vi "get_numbers_in_string.vi"(3 "String":string="one 2 -3 4.0 5.5") -> (0 "Total numbers":i32, 1 "Extracted Numbers":dbl[](array[numeric]) format="%#.6g")   [LabVIEW 2018]
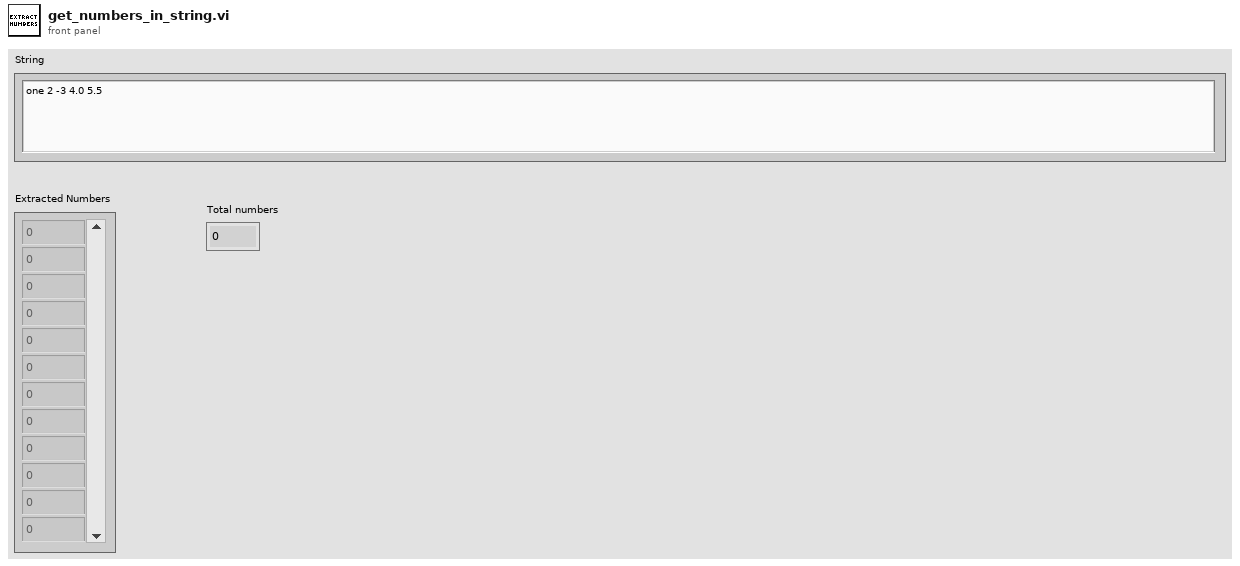
[diagram p1: front panel]
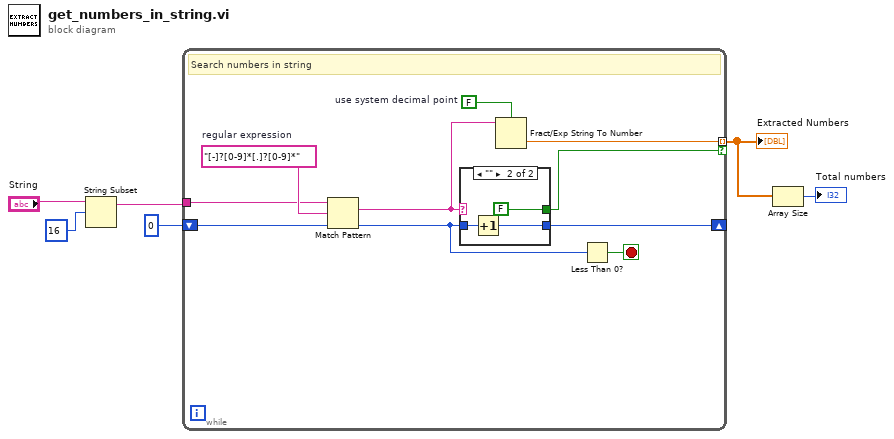
[diagram p0: block diagram]
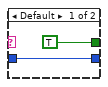
[diagram p2: hidden frame]
diagram:
  n1 = String Subset(string="String", offset (0)=16) -> (substring=w2:string)  [unwired: 1 in]
  n2 = while {
    shift-left: 0 -> [w12]
    shift-right: [w7] -> _
    tunnel: [w16] -> w5 mode=indexing if=w9
    tunnel: w2 -> [w11]
    stop <- w15 stop-if-true
    w14 = FALSE  # use system decimal point
    w13 = "[-]?[0-9]*[.]?[0-9]*"  # regular expression
    # "Search numbers in string"
    n3 = Match Pattern(string=w11, regular expression=w13, offset (0)=w12) -> (match substring=w10:string, offset past match=w8:i32)  [unwired: 2 out]
    n4 = case shown="\"\"" w10 {
      tunnel: [w18 w20] -> w7
      tunnel: [TRUE FALSE] -> w9
      tunnel: w8 -> [w18 w21]
      frame Default {
      }
      frame "" {
        n5 = Increment(x=w21) -> (x+1=w20:i32)
      }
    }
    n6 = Fract/Exp String To Number(use system decimal point (T)=w14, string=w10) -> (number=w16:dbl)  [unwired: 2 in, 1 out]
    n7 = Less Than 0?(x=w8) -> (x < 0?=w15:bool)
  }
  "Extracted Numbers" <- w5
  n8 = Array Size(array=w5) -> (size(s)=→"Total numbers":i32)
